vi "Create ForecastData Waveforms.vi"(9 "ForecastData Array":T1[](array[typedef]), 11 "Measured Powers":dbl[](array[numeric])) -> (3 "Forecast Waveforms Array":waveform(dbl)[](array[waveform]))   [LabVIEW 2018, in "Generic Optimization Actor.lvlib" / "Generic Optimization.lvclass"]
doc: "Replaces first element of forecast with measured value and then converts the forecast into a waveform."
uses:
  Generic Optimization.lvclass
  <vilib>/ORNL/CSEISMIC DDS/CSEISMIC DDS Base/Data Types/ForecastData_Data.ctl
  <vilib>/ORNL/CSEISMIC DDS/CSEISMIC DDS Base/Data Types/Controls/DeviceID.ctl
  <vilib>/ORNL/CSEISMIC DDS/CSEISMIC DDS Base/CSEISMIC DDS.lvclass
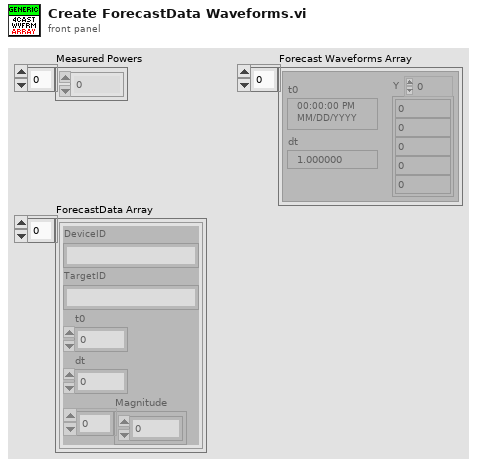
[diagram p1: front panel]
types:
  T1 = typedef "CSEISMIC DDS.lvlib/CSEISMIC DDS.lvclass/ForecastData_Data.ctl" = cluster{"DeviceID":T2, "TargetID":T2, "t0":dbl, "dt":dbl, "Magnitude":dbl[]}
  T2 = typedef "CSEISMIC DDS.lvlib/CSEISMIC DDS.lvclass/DeviceID.ctl" = string
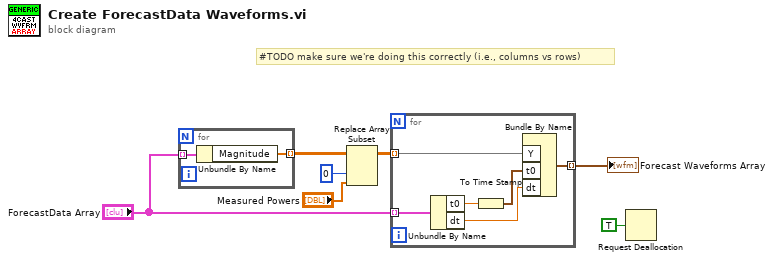
[diagram p0: block diagram]
diagram:
  # "#TODO make sure we're doing this correctly (i.e., columns vs rows)"
  n1 = for {
    tunnel: "ForecastData Array" -> [w9] mode=indexing
    tunnel: [w8] -> w2 mode=indexing
    n2 = Unbundle By Name(w9) -> ("Magnitude"=w8:dbl[])
  }
  n3 = Replace Array Subset(array=w2, new element="Measured Powers", index (col)=0 ("disabled index (col)")) -> (w6:dbl[][])  [unwired: 1 in]
  n4 = for {
    tunnel: w6 -> [w11] mode=indexing
    tunnel: "ForecastData Array" -> [w15] mode=indexing
    tunnel: [w10] -> w7 mode=indexing
    n5 = Unbundle By Name(w15) -> ("t0"=w13:dbl, "dt"=w14:dbl)
    n6 = To Time Stamp(1:w13) -> (0:w12:timestamp)
    n7 = Bundle By Name("Y"=w11, "t0"=w12, "dt"=w14) -> (w10:waveform(dbl))  [unwired: 1 in]
  }
  "Forecast Waveforms Array" <- w7
  n8 = Request Deallocation(TRUE ("flag")) -> ()
